vi "Database.GetTimeOfLatestFileChange.vi"(9 "Ref":string, 10 "System":string, 11 "VariantsFolder":path) -> (2 "Time Stamp":timestamp, 3 "FilePath":path)   [LabVIEW 2016]
uses:
  <vilib>/regexp/Match Regular Expression.xnode
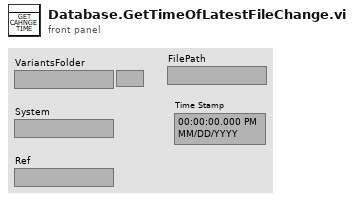
[diagram p1: front panel]
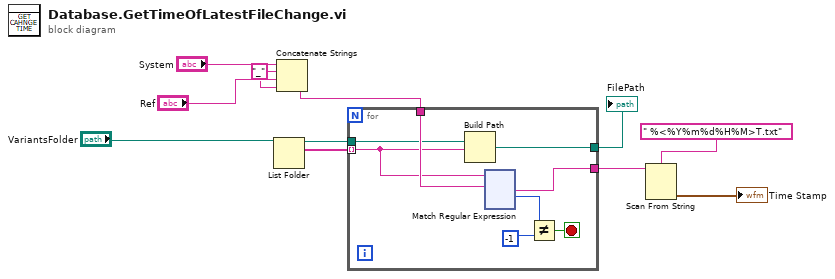
[diagram p0: block diagram]
diagram:
  w1 = "_" ("string")
  n1 = List Folder(path="VariantsFolder") -> (path out=w3:path, filenames=w5:string[])  [unwired: 3 in, 2 out]
  n2 = Concatenate Strings("System", w1, "Ref", w1) -> (w8:string)
  n3 = for {
    tunnel: w5 -> [w13] mode=indexing
    tunnel: w8 -> [w19]
    tunnel: [w18] -> w10
    tunnel: w3 -> [w14]
    tunnel: [w12] -> w2
    stop <- w17 stop-if-true
    n4 = Build Path(base path=w14, name or relative path=w13) -> (appended path=w12:path)
    n5 = xnode "Match Regular Expression"("input string"=w13, "regular expression"=w19) -> ("after match"=w18:string, "offset past match"=w15:i32)  [unwired: 4 in, 3 out]
    n6 = Not Equal?(x=w15, y=-1) -> (x != y?=w17:bool)
  }
  "FilePath" <- w2
  n7 = Scan From String(format string=" %<%Y%m%d%H%M>T.txt", input string=w10) -> (output 1=→"Time Stamp":timestamp)  [unwired: 3 in, 3 out]
